vi "AO array setup.vi"(0 "DAC Array":T1(array[cluster])=[{"start voltage (V)"=5.0, "start time (ms)"=0.0, "Enable DAC"=TRUE, "Hinge points"=[{"time (ms)"=1.0, "voltage (V)"=3.0, "transition"=2, "tau"=5.0, "asymptote"=0.0, "end time"=0.0}, {"time (ms)"=10.0, "voltage (V)"=1.0, "transition"=2, "tau"=3.0, "asymptote"=0.0, "end time"=0.0}]}, {"start voltage (V)"=-3.5, "start time (ms)"=0.0, "Enable DAC"=FALSE, "Hinge points"=[{"time (ms)"=400.0, "voltage (V)"=-3.5, "transition"=0, "tau"=0.0, "asymptote"=0.0, "end time"=401.0}, {"time (ms)"=500.0, "voltage (V)"=-2.5, "transition"=1, "tau"=0.0, "asymptote"=0.0, "end time"=501.0}]}, {"start voltage (V)"=-3.55, "start time (ms)"=0.0, "Enable DAC"=FALSE, "Hinge points"=[{"time (ms)"=4500.0, "voltage (V)"=0.0, "transition"=0, "tau"=0.0, "asymptote"=0.0, "end time"=4501.0}]}, {"start voltage (V)"=0.0, "start time (ms)"=0.0, "Enable DAC"=FALSE, "Hinge points"=[]}, {"start voltage (V)"=-5.0, "start time (ms)"=0.0, "Enable DAC"=FALSE, "Hinge points"=[]}, {"start voltage (V)"=0.0, "start time (ms)"=0.0, "Enable DAC"=FALSE, "Hinge points"=[]}, {"start voltage (V)"=0.0, "start time (ms)"=0.0, "Enable DAC"=FALSE, "Hinge points"=[]}, {"start voltage (V)"=0.0, "start time (ms)"=0.0, "Enable DAC"=FALSE, "Hinge points"=[]}] {"start voltage (V)" format="%.4f"; "start time (ms)" format="%.3f"; "Hinge points"."transition" items=["Step", "Ramp", "Exp"]; "Hinge points"."voltage (V)" format="%.4f"; "Hinge points"."time (ms)" format="%.3f"}, 1 "pre-evap time step (ms)":dbl=1.0 format="%.3f") -> (2 "Output Array":waveform(dbl)[](array[waveform])=[{"t0"=timestamp(0 s since 1904-01-01), "dt"=0.001, "Y"=[5.0, 5.0, 4.093653765389909, 3.3516002301781964, 3.0, 3.0, 3.0, 3.0, 3.0, 3.0, 2.4940375810397097, 1.7870560165626665, 1.2804815896164226, 1.0]}, {"t0"=timestamp(0 s since 1904-01-01), "dt"=0.001, "Y"=[-3.5, -3.5, -3.5, -3.5, -3.5, -3.5, -3.5, -3.5, -3.5, -3.5, -3.5, -3.5, -3.5, -3.5, -3.5]}, {"t0"=timestamp(0 s since 1904-01-01), "dt"=0.001, "Y"=[-3.55, -3.55, -3.55, -3.55, -3.55, -3.55, -3.55, -3.55, -3.55, -3.55, -3.55, -3.55, -3.55, -3.55, -3.55]}, {"t0"=timestamp(0 s since 1904-01-01), "dt"=0.001, "Y"=[0.0, 0.0, 0.0, 0.0, 0.0, 0.0, 0.0, 0.0, 0.0, 0.0, 0.0, 0.0, 0.0, 0.0, 0.0]}, {"t0"=timestamp(0 s since 1904-01-01), "dt"=0.001, "Y"=[-5.0, -5.0, -5.0, -5.0, -5.0, -5.0, -5.0, -5.0, -5.0, -5.0, -5.0, -5.0, -5.0, -5.0, -5.0]}, {"t0"=timestamp(0 s since 1904-01-01), "dt"=0.001, "Y"=[0.0, 0.0, 0.0, 0.0, 0.0, 0.0, 0.0, 0.0, 0.0, 0.0, 0.0, 0.0, 0.0, 0.0, 0.0]}, {"t0"=timestamp(0 s since 1904-01-01), "dt"=0.001, "Y"=[0.0, 0.0, 0.0, 0.0, 0.0, 0.0, 0.0, 0.0, 0.0, 0.0, 0.0, 0.0, 0.0, 0.0, 0.0]}, {"t0"=timestamp(0 s since 1904-01-01), "dt"=0.001, "Y"=[0.0, 0.0, 0.0, 0.0, 0.0, 0.0, 0.0, 0.0, 0.0, 0.0, 0.0, 0.0, 0.0, 0.0, 0.0]}], 3 "ntimes":u32, 4 "DAC Array out":T1(array[cluster])=[{"start voltage (V)"=5.0, "start time (ms)"=0.0, "Enable DAC"=TRUE, "Hinge points"=[{"time (ms)"=1.0, "voltage (V)"=3.0, "transition"=2, "tau"=5.0, "asymptote"=0.0, "end time"=5.0}, {"time (ms)"=10.0, "voltage (V)"=1.0, "transition"=2, "tau"=3.0, "asymptote"=0.0, "end time"=14.0}]}, {"start voltage (V)"=-3.5, "start time (ms)"=0.0, "Enable DAC"=FALSE, "Hinge points"=[{"time (ms)"=400.0, "voltage (V)"=-3.5, "transition"=0, "tau"=0.0, "asymptote"=0.0, "end time"=0.0}, {"time (ms)"=500.0, "voltage (V)"=-2.5, "transition"=1, "tau"=0.0, "asymptote"=0.0, "end time"=0.0}]}, {"start voltage (V)"=-3.55, "start time (ms)"=0.0, "Enable DAC"=FALSE, "Hinge points"=[{"time (ms)"=4500.0, "voltage (V)"=0.0, "transition"=0, "tau"=0.0, "asymptote"=0.0, "end time"=0.0}]}, {"start voltage (V)"=0.0, "start time (ms)"=0.0, "Enable DAC"=FALSE, "Hinge points"=[]}, {"start voltage (V)"=-5.0, "start time (ms)"=0.0, "Enable DAC"=FALSE, "Hinge points"=[]}, {"start voltage (V)"=0.0, "start time (ms)"=0.0, "Enable DAC"=FALSE, "Hinge points"=[]}, {"start voltage (V)"=0.0, "start time (ms)"=0.0, "Enable DAC"=FALSE, "Hinge points"=[]}, {"start voltage (V)"=0.0, "start time (ms)"=0.0, "Enable DAC"=FALSE, "Hinge points"=[]}])   [LabVIEW 2017]
doc: "This subVI sets up the AO (analog output) array to send to the board."
uses:
  <vilib>/Waveform/WDTOps.llb/WDT Waveform Duration DBL.vi
panel:
  out "Array 2":dbl[](array[numeric])
  out "Array":waveform(dbl)[](array[waveform])
  out "Temp Waveform 4":waveform(dbl)={"t0"=timestamp(0 s since 1904-01-01), "dt"=0.001, "Y"=[5.0, 5.0, 4.093653765389909, 3.3516002301781964, 3.0, 3.0, 3.0, 3.0, 3.0, 3.0, 2.4940375810397097, 1.7870560165626665, 1.2804815896164226, 1.0]}
  out "max time (ms)":dbl=14.0 format="%.2f"
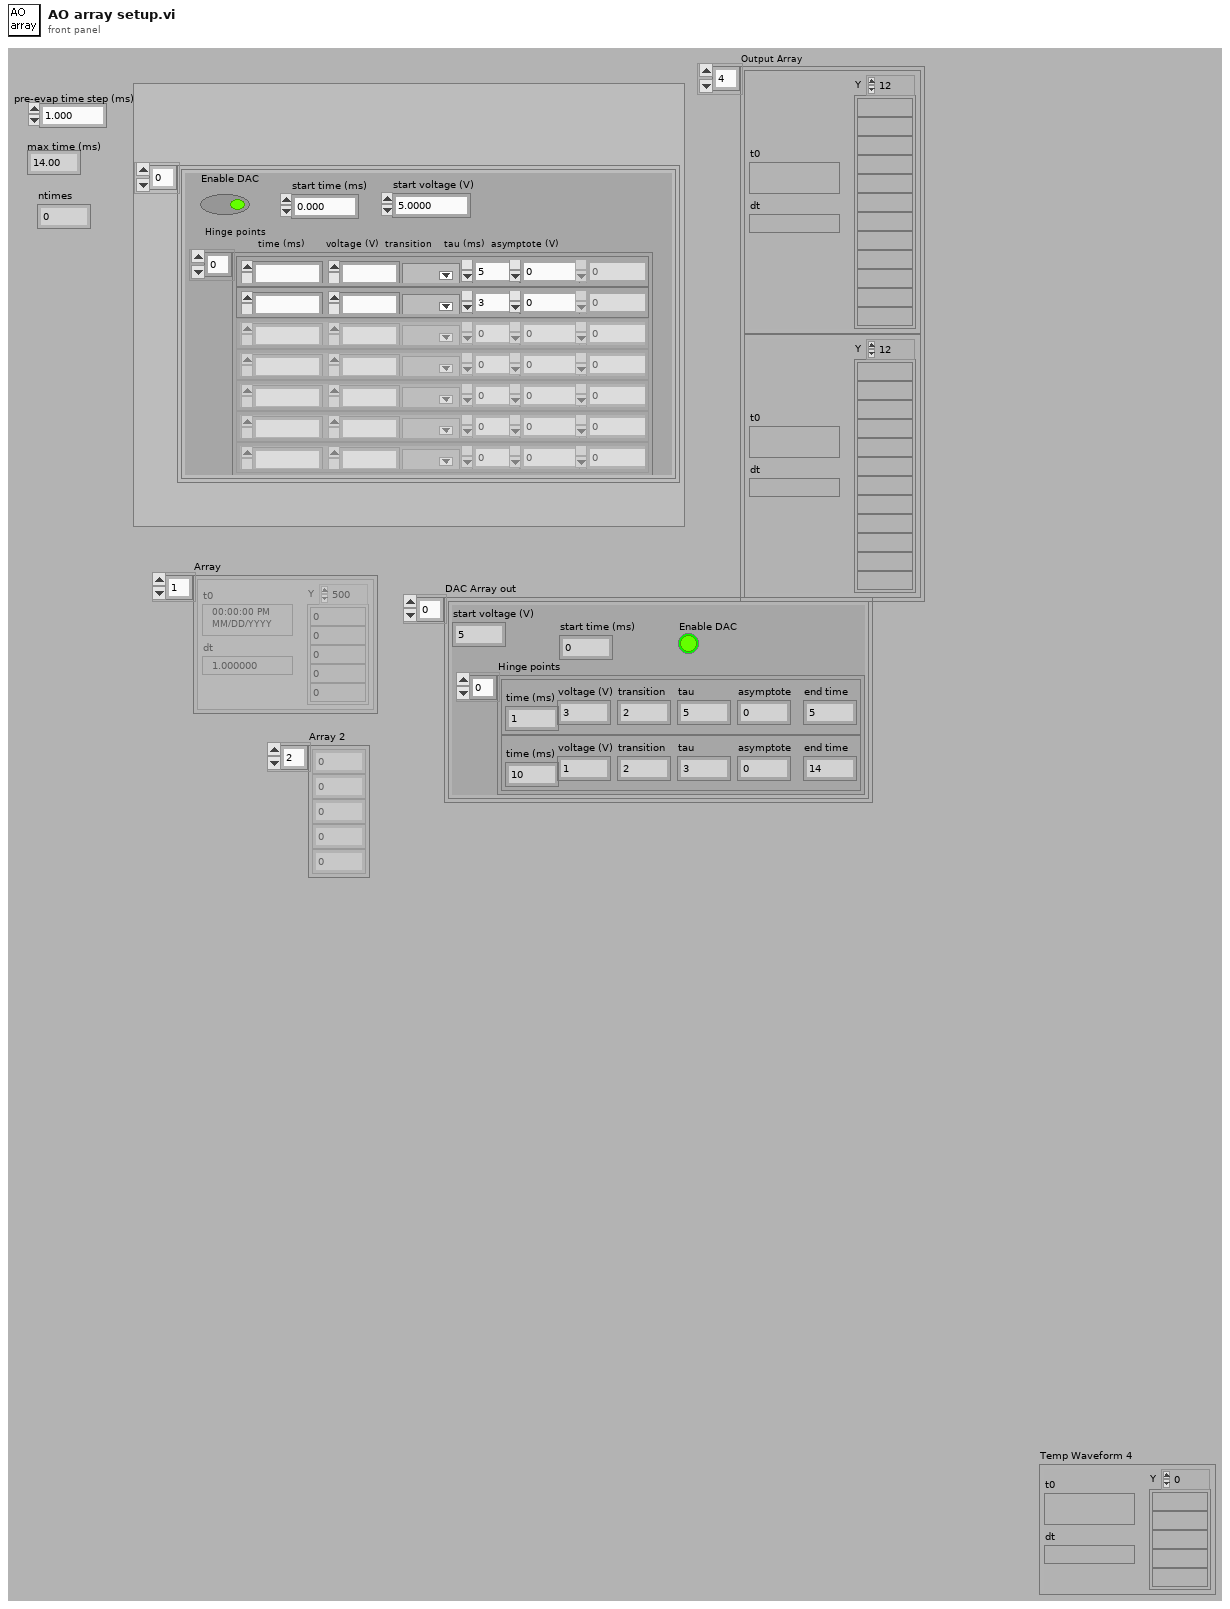
[diagram p1: front panel]
types:
  T1 = cluster{"start voltage (V)":dbl, "start time (ms)":dbl, "Enable DAC":bool, "Hinge points":cluster{"time (ms)":dbl, "voltage (V)":dbl, "transition":u16, "tau":dbl, "asymptote":dbl, "end time":dbl}[]}[]
  T2 = cluster{"time (ms)":dbl, "voltage (V)":dbl, "transition":u16, "tau":dbl, "asymptote":dbl, "end time":dbl}[]
  T3 = cluster{"time (ms)":dbl, "voltage (V)":dbl, "transition":u16, "tau":dbl, "asymptote":dbl, "end time":dbl}
  T4 = cluster{"start voltage (V)":dbl, "start time (ms)":dbl, "Enable DAC":bool, "Hinge points":cluster{"time (ms)":dbl, "voltage (V)":dbl, "transition":u16, "tau":dbl, "asymptote":dbl, "end time":dbl}[]}
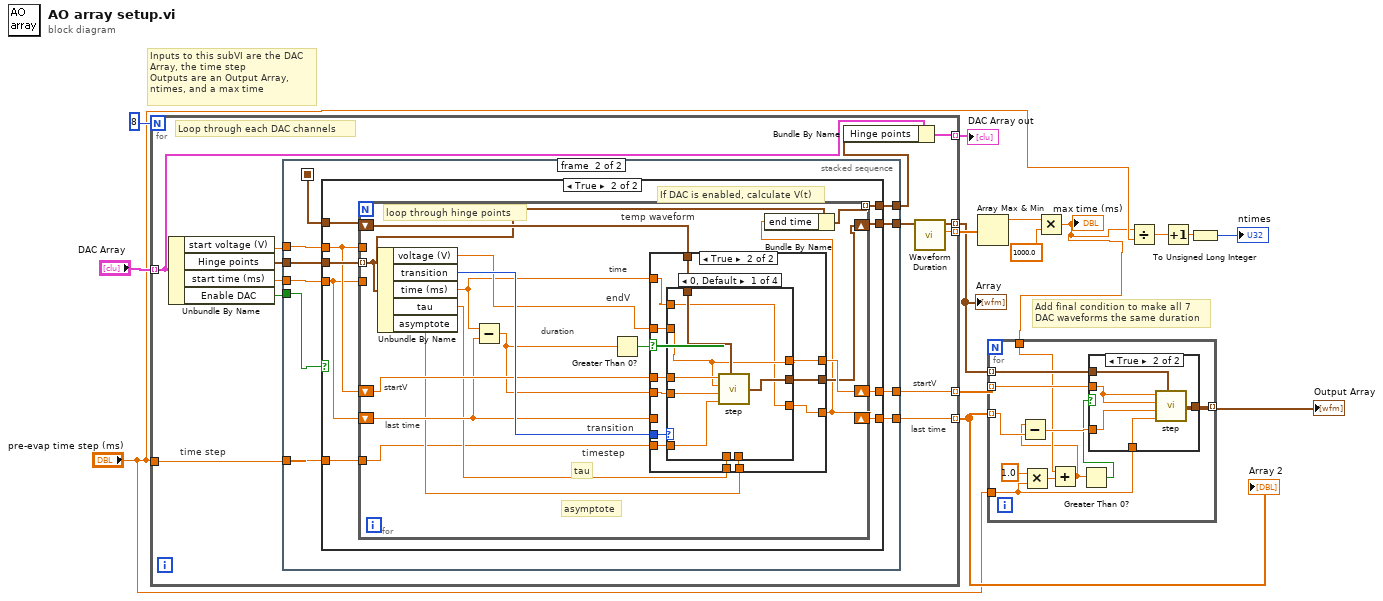
[diagram p0: block diagram]
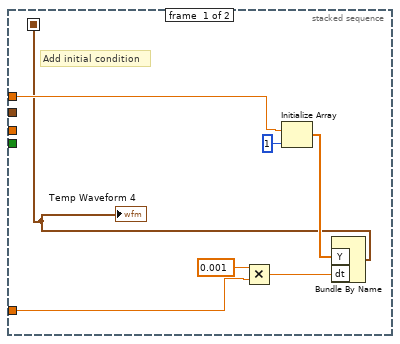
[diagram p3: hidden frame]
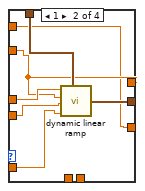
[diagram p6: hidden frame]
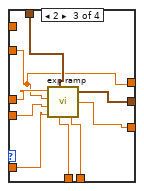
[diagram p7: hidden frame]
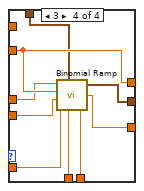
[diagram p8: hidden frame]
diagram:
  # "Add final condition to make all 7 DAC waveforms the same duration"
  # "Inputs to this subVI are the DAC Array, the time step\nOutputs are an Output Array, ntimes, and a max time"
  n1 = for {
    N: 8 -> [_]
    tunnel: "DAC Array" -> [w18] mode=indexing
    tunnel: "pre-evap time step (ms)" -> [w26]
    tunnel: [w22] -> w13 mode=indexing
    tunnel: [w21] -> w11 mode=indexing
    tunnel: [w20] -> w12 mode=indexing
    tunnel: [w19] -> w10 mode=indexing
    tunnel: [w17] -> w7 mode=indexing
    # "Loop through each DAC channels"
    # "startV"
    # "last time"
    # "time step"
    n2 = Unbundle By Name(w18) -> ("start voltage (V)"=w27:dbl, "Hinge points"=w24:T2, "start time (ms)"=w28:dbl, "Enable DAC"=w25:bool)
    n3 = stacked-sequence {
      seq-local: [w29 _] -> [_ w40]
      tunnel: w24 -> [_ w45]
      tunnel: w28 -> [_ w44]
      tunnel: w27 -> [w31 w43]
      tunnel: w26 -> [w30 w42]
      tunnel: w25 -> [_ w41]
      tunnel: [_ w39] -> w23
      tunnel: [_ w38] -> w20
      tunnel: [_ w37] -> w21
      tunnel: [_ w36] -> w16
      frame #0 {
        # "Add initial condition"
        n4 = Multiply(x=0.001 ("y"), y=w30) -> (x*y=w34:dbl)
        n5 = Initialize Array(w31, 1 ("Dimension Size")) -> (w32:dbl[])
        n6 = Bundle By Name("Y"=w32, "dt"=w34) -> (w29:waveform(dbl))  [unwired: 1 in]
        "Temp Waveform 4" <- w29
      }
      frame #1 {
        n7 = case shown="True" w41 {
          tunnel: w45 -> [w46 w58]
          tunnel: w44 -> [w48 w54]
          tunnel: w43 -> [w49 w55]
          tunnel: w42 -> [_ w57]
          tunnel: w40 -> [w47 w56]
          tunnel: [w47 w53] -> w39
          tunnel: [w49 w52] -> w38
          tunnel: [w48 w51] -> w37
          tunnel: [w46 w50] -> w36
          frame False {
          }
          frame True {
            # "If DAC is enabled, calculate V(t)"
            n8 = for {
              tunnel: w58 -> [w61] mode=indexing
              tunnel: w54 -> [_]
              tunnel: w55 -> [_]
              tunnel: w57 -> [w63]
              shift-right: [w62] -> w53
              shift-left: w56 -> [w71]
              shift-right: [w68] -> w52
              shift-left: w55 -> [w70]
              shift-right: [w59] -> w51
              shift-left: w54 -> [w67]
              tunnel: [w60] -> w50 mode=indexing
              # "transition"
              # "tau"
              # "asymptote"
              # "temp waveform"
              # "time"
              # "last time"
              # "duration"
              # "timestep"
              # "endV"
              # "startV"
              # "loop through hinge points"
              n9 = Unbundle By Name(w61) -> ("voltage (V)"=w72:dbl, "transition"=w73:u16, "time (ms)"=w66:dbl, "tau"=w65:dbl, "asymptote"=w64:dbl)
              n10 = Subtract(x=w66, y=w67) -> (x-y=w69:dbl)
              n11 = Greater Than 0?(x=w69) -> (x > 0?=w74:bool)
              n12 = case shown="True" w74 {
                tunnel: w69 -> [_ w89]
                tunnel: [w75 w88] -> w62
                tunnel: w73 -> [_ w87]
                tunnel: w72 -> [_ w86]
                tunnel: w63 -> [_ w85]
                tunnel: w71 -> [w75 w84]
                tunnel: w70 -> [w77 w83]
                tunnel: [w77 w82] -> w68
                tunnel: w67 -> [w76 _]
                tunnel: [w76 w78] -> w59
                tunnel: w66 -> [_ w79]
                tunnel: w65 -> [_ w81]
                tunnel: w64 -> [_ w80]
                frame False {
                }
                frame True {
                  n13 = case shown="0, Default" w87 {
                    tunnel: w89 -> [w95 w102 w106 w119]
                    tunnel: [w96 w103 w112 w113] -> w88
                    tunnel: w86 -> [w91 w98 w105 w121]
                    tunnel: w85 -> [w94 w100 w109 w118]
                    tunnel: w84 -> [w93 w101 w111 w114]
                    tunnel: w83 -> [w92 w99 w110 w120]
                    tunnel: [w91 w98 w105 w121] -> w82
                    tunnel: w81 -> [_ _ w108 w117]
                    tunnel: w80 -> [_ _ w107 w116]
                    tunnel: [w90 w97 w104 w115] -> w78
                    tunnel: w79 -> [w90 w97 _ _]
                    frame 0, Default {
                      n14 = call "step.vi"("start"=w92, "end"=w91, "duration"=w95, "time step (ms)"=w94, "input waveform"=w93) -> ("waveform out"=w96:waveform(dbl))
                    }
                    frame 1 {
                      n15 = call "dynamic linear ramp.vi"("start"=w99, "end"=w98, "duration"=w102, "time step (ms)"=w100, "input waveform"=w101) -> ("waveform out"=w103:waveform(dbl))
                    }
                    frame 2 {
                      n16 = call "exp ramp.vi"("start"=w110, "input waveform"=w111, "end"=w105, "hold before ramp"=w106, "tau (ms)"=w108, "time step (ms)"=w109, "asymptote"=w107) -> ("waveform out"=w112:waveform(dbl), "end time (ms)"=w104:dbl)
                    }
                    frame 3 {
                      n17 = call "Binomial Ramp.vi"("start"=w120, "input waveform"=w114, "end"=w121, "hold before ramp"=w119, "tau (ms)"=w117, "time step (ms)"=w118, "asymptote"=w116) -> ("waveform out"=w113:waveform(dbl), "end time (ms)"=w115:dbl)
                    }
                  }
                }
              }
              n18 = Bundle By Name(cluster=w61, "end time"=w59) -> (w60:T3)
            }
          }
        }
      }
    }
    n19 = Bundle By Name(cluster=w18, "Hinge points"=w16) -> (w17:T4)
    n20 = call-poly <vilib>:"Waveform Duration.vi"("waveform in"=w23) -> ("duration"=w22:dbl, "waveform out"=w19:waveform(dbl))  [unwired: 8 in, 1 out]
  }
  "DAC Array out" <- w7
  "Array" <- w10
  "Array 2" <- w11
  n21 = Array Max & Min(array=w13) -> (max value=w8:dbl)  [unwired: 3 out]
  n22 = Multiply(x=w8, y=1000.0) -> (x*y=w1:dbl)
  "max time (ms)" <- w1
  n23 = for {
    tunnel: w12 -> [w130] mode=indexing
    tunnel: w11 -> [w129] mode=indexing
    tunnel: w10 -> [w132] mode=indexing
    tunnel: [w131] -> w9 mode=indexing
    tunnel: "pre-evap time step (ms)" -> [w125]
    tunnel: w1 -> [w123]
    n24 = Multiply(x=1.0 ("y"), y=w125) -> (x*y=w127:dbl)
    n25 = Add(x=w123, y=w127) -> (x+y=w122:dbl)
    n26 = Subtract(x=w122, y=w129) -> (x-y=w128:dbl)
    n27 = Greater Than 0?(x=w122) -> (x > 0?=w124:bool)
    n28 = case shown="True" w124 {
      tunnel: w132 -> [w133 w138]
      tunnel: [w133 w137] -> w131
      tunnel: w130 -> [_ w136]
      tunnel: w125 -> [_ w135]
      tunnel: w128 -> [_ w134]
      frame False {
      }
      frame True {
        n29 = call "step.vi"("start"=w136, "end"=w136, "duration"=w134, "time step (ms)"=w135, "input waveform"=w138) -> ("waveform out"=w137:waveform(dbl))
      }
    }
  }
  "Output Array" <- w9
  n30 = Divide(x=w1, y="pre-evap time step (ms)") -> (x/y=w5:dbl)
  n31 = Increment(x=w5) -> (x+1=w4:dbl)
  n32 = To Unsigned Long Integer(number=w4) -> (unsigned 32bit integer=→"ntimes":u32)
